vi "rid_to_path.vi"(10 "RID":string=".chmx_2", 11 "Base":path[](array[path])=[path "D:/Data/2014/06/28/20140628_162708", path "Z:/Data/2014/06/28/20140628_162708"]) -> (2 "Paths":path[](array[path]))   [LabVIEW 2013]
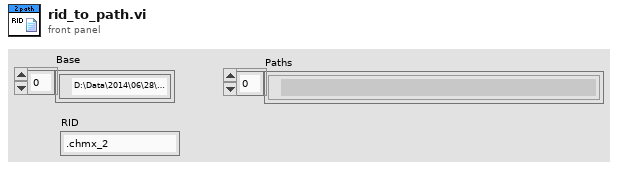
[diagram p1: front panel]
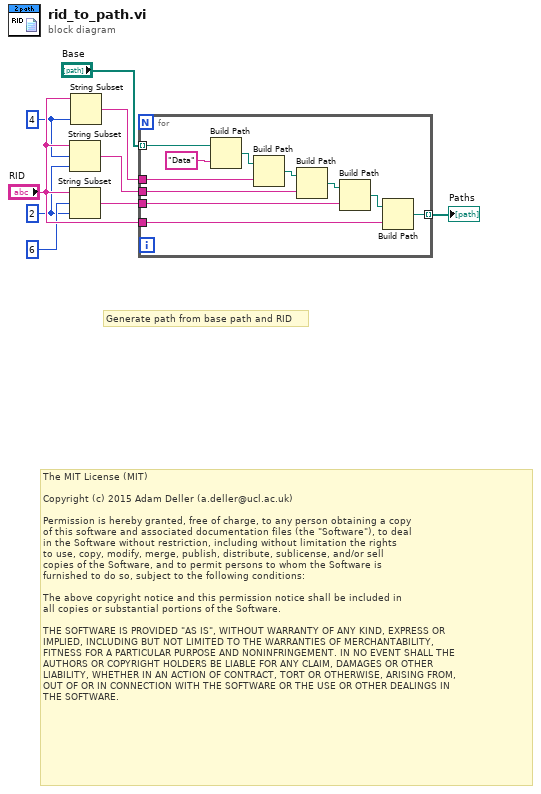
[diagram p0: block diagram]
diagram:
  w3 = 4 ("offset (0)")
  w1 = 2 ("length (rest)")
  # "The MIT License (MIT)\n\nCopyright (c) 2015 Adam Deller (a.deller@ucl.ac.uk) \n\nPermission is hereby granted, free of charge, to any person obtaining a copy\nof this software and associated documentation files (the \"Software\"), to deal\nin the Software without restriction, including without limitation the rights\nto use, copy, modify, merge, publish, distribute, sublicense, and/or sell\ncopies of the Software, and to permit persons to whom the Software is\nfurnished to do so, subject to the following conditions:\n\nThe above copyright notice and this permission notice shall be included in\nall copies or substantial portions of the Software.\n\nTHE SOFTWARE IS PROVIDED \"AS IS\", WITHOUT WARRANTY OF ANY KIND, EXPRESS OR\nIMPLIED, INCLUDING BUT NOT LIMITED TO THE WARRANTIES OF MERCHANTABILITY,\nFITNESS FOR A PARTICULAR PURPOSE AND NONINFRINGEMENT. IN NO EVENT SHALL THE\nAUTHORS OR COPYRIGHT HOLDERS BE LIABLE FOR ANY CLAIM, DAMAGES OR OTHER\nLIABILITY, WHETHER IN AN ACTION OF CONTRACT, TORT OR OTHERWISE, ARISING FROM,\nOUT OF OR IN CONNECTION WITH THE SOFTWARE OR THE USE OR OTHER DEALINGS IN\nTHE SOFTWARE."
  # "Generate path from base path and RID"
  n1 = String Subset(string="RID", offset (0)=w3, length (rest)=w1) -> (substring=w7:string)
  n2 = String Subset(string="RID", offset (0)=6, length (rest)=w1) -> (substring=w6:string)
  n3 = String Subset(string="RID", length (rest)=w3) -> (substring=w8:string)  [unwired: 1 in]
  n4 = for {
    tunnel: "Base" -> [w18] mode=indexing
    tunnel: w8 -> [w20]
    tunnel: w7 -> [w15]
    tunnel: w6 -> [w14]
    tunnel: "RID" -> [w11]
    tunnel: [w10] -> w4 mode=indexing
    n5 = Build Path(base path=w18, name or relative path="Data") -> (appended path=w17:path)
    n6 = Build Path(base path=w17, name or relative path=w20) -> (appended path=w16:path)
    n7 = Build Path(base path=w16, name or relative path=w15) -> (appended path=w13:path)
    n8 = Build Path(base path=w13, name or relative path=w14) -> (appended path=w12:path)
    n9 = Build Path(base path=w12, name or relative path=w11) -> (appended path=w10:path)
  }
  "Paths" <- w4
